vi "Update Setpoint.vi"(8 "error in (no error)":errorcluster, 11 "Sensor & Control in":refnum<class "Sensor & Control.lvclass">) -> (0 "error out":errorcluster, 3 "Sensor & Control out":refnum<class "Sensor & Control.lvclass">)   [LabVIEW 2013, in "Sensor & Control.lvlib" / "Sensor & Control.lvclass"]
uses:
  Sensor & Control.lvclass
  Sensor & Control.lvclass/Sensor & Control.ctl
  Read Setpoint.vi
  PluginInterface/PluginInterface.lvlibp/PluginInterfaceClass/Read Name.vi
  PluginInterface/PluginInterface.lvlibp/PluginInterfaceClass/Read DVR.vi
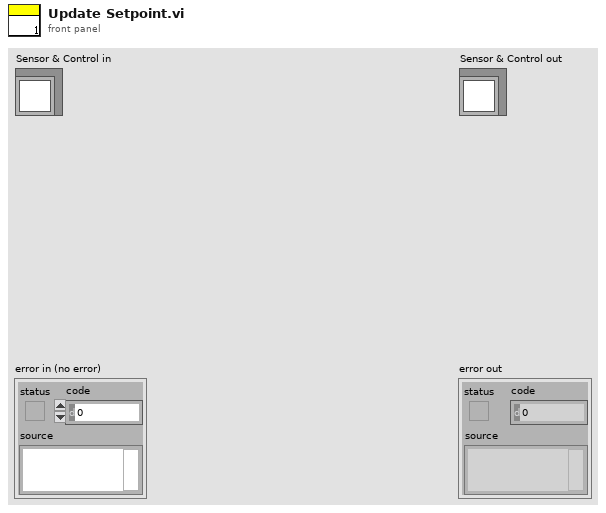
[diagram p1: front panel]
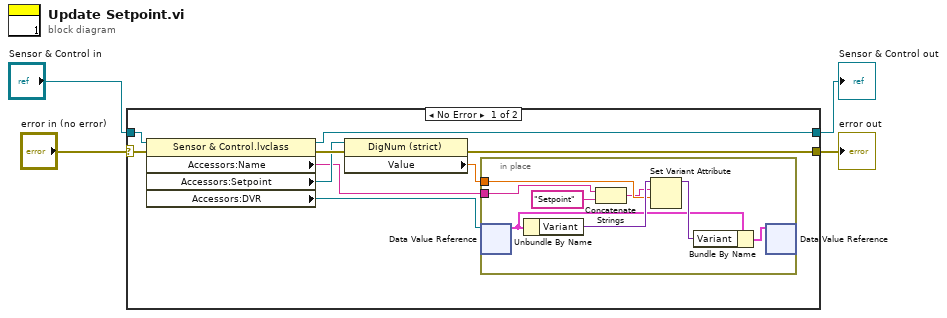
[diagram p0: block diagram]
diagram:
  n1 = case shown="No Error" "error in (no error)" {
    selector: "error in (no error)" -> [w11 w23]
    tunnel: [w5 w23] -> w1
    tunnel: [w6 w22] -> w2
    tunnel: "Sensor & Control in" -> [w10 w22]
    frame No Error {
      n2 = property class="Sensor & Control.lvclass"(reference=w10, error in=w11) -> (reference out=w6:refnum<class "Sensor & Control.lvclass">, error out=w13:errorcluster, "Accessors:Name"=w7:string, "Accessors:Setpoint"=w8:refnum<vi>, "Accessors:DVR"=w12:refnum<data-value>)
      n3 = property class="DigNum (strict)"(reference=w8, error in=w13) -> (error out=w5:errorcluster, "Value"=w9:dbl)  [unwired: 1 out]
      n4 = in-place {
        in-place-border: w9 -> [w17]
        in-place-border: w7 -> [w15]
        n5 = in-place-dvr #1(w12) -> (w18:cluster{"Array":string[], "Variant":variant})  [unwired: 1 out]
        n6 = Unbundle By Name(w18) -> ("Variant"=w20:variant)
        n7 = Concatenate Strings(w15, "Setpoint") -> (w14:string)
        n8 = Set Variant Attribute(Variant=w20, name=w14, value=w17) -> (Variant out=w19:variant)  [unwired: 1 in, 2 out]
        n9 = Bundle By Name(cluster=w18, "Variant"=w19) -> (w21:cluster{"Array":string[], "Variant":variant})
        n10 = in-place-dvr #1(w21) -> ()  [unwired: 2 out]
      }
    }
    frame Error {
    }
  }
  "error out" <- w1
  "Sensor & Control out" <- w2
